vi "Read Metadata from SnP File.vi"(0 "SnP File Path in":path, 5 "Key":string, 11 "error in (no error)":errorcluster) -> (4 "SnP File Path out":path, 6 "Value":string, 15 "error out":errorcluster)   [LabVIEW 2023, in "RFFixtureCharact.RFPM.lvlib" / "Charact Result Accessor.lvclass"]
uses:
  Charact Result Accessor.lvclass
  Global IDs.vi
  <vilib>/regexp/Match Regular Expression.xnode
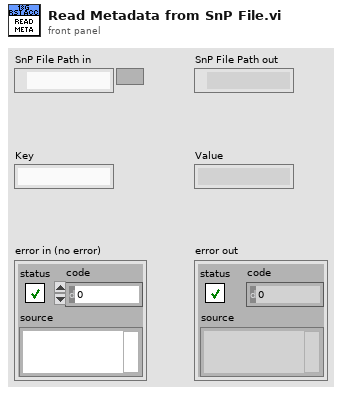
[diagram p1: front panel]
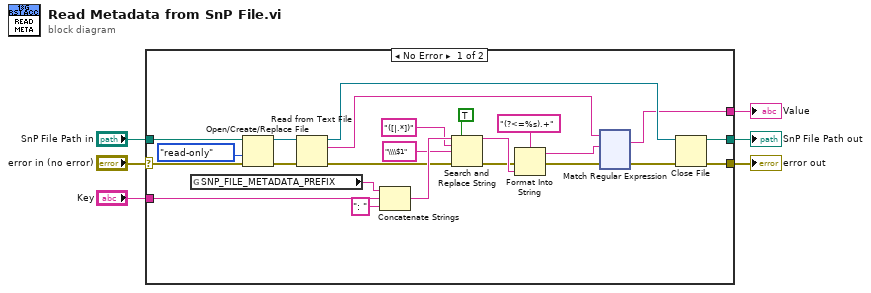
[diagram p0: block diagram]
diagram:
  n1 = case shown="No Error" "error in (no error)" {
    selector: "error in (no error)" -> [w22 w149]
    tunnel: [w30 w149] -> w5
    tunnel: "SnP File Path in" -> [w23 w148]
    tunnel: [w29 w148] -> w3
    tunnel: [w14 _] -> w2
    tunnel: "Key" -> [w17 _]
    frame No Error {
      n2 = global read "Global IDs.vi" "SNP_FILE_METADATA_PREFIX"() -> (w18:string)
      n3 = Open/Create/Replace File(file path (use dialog)=w23, error in=w22, access (0:read/write)=enum16{"read/write", "read-only", "write-only"}."read-only") -> (refnum out=w21:refnum<file>, error out=w20:errorcluster)  [unwired: 3 in, 1 out]
      n4 = Read from Text File(file (use dialog)=w21, error in=w20) -> (refnum out=w24:refnum<file>, text=w28:string, error out=w8:errorcluster)  [unwired: 2 in, 1 out]
      n5 = Concatenate Strings(w18, w17, ": " ("string")) -> (w13:string)
      n6 = Search and Replace String(replace all?=TRUE ("replace all? (F)"), input string=w13, search string="([|.*])", replace string="\\\\$1" ("replace string (\"\")"), error in=w8) -> (result string=w10:string, error out=w7:errorcluster)  [unwired: 3 in, 2 out]
      n7 = Format Into String(format string="(?<=%s).+" ("regular expression"), error in=w7, w10) -> (resulting string=w25:string, error out=w26:errorcluster)  [unwired: 1 in]
      n8 = xnode "Match Regular Expression"("input string"=w28, "regular expression"=w25, "error in"=w26) -> ("whole match"=w14:string, "error out"=w15:errorcluster)  [unwired: 3 in, 3 out]
      n9 = Close File(refnum=w24, error in=w15) -> (path=w29:path, error out=w30:errorcluster)
    }
    frame Error {
    }
  }
  "error out" <- w5
  "SnP File Path out" <- w3
  "Value" <- w2
